vi "Field Draw Field(circular).vi"(6 "Lado,radius, stretch":i32[](array[numeric]), 8 "new picture in":picture, 9 "Offset":cluster{"Width":dbl, "Height":dbl}, 10 "Scale":dbl, 11 "Field Size":T2) -> (0 "new picture out":picture, 1 "Offset Out":cluster{"Width":dbl, "Height":dbl}, 2 "Scale Out":dbl)   [LabVIEW 2017]
panel:
  in  "left":i16=1
  in  "rect":T1
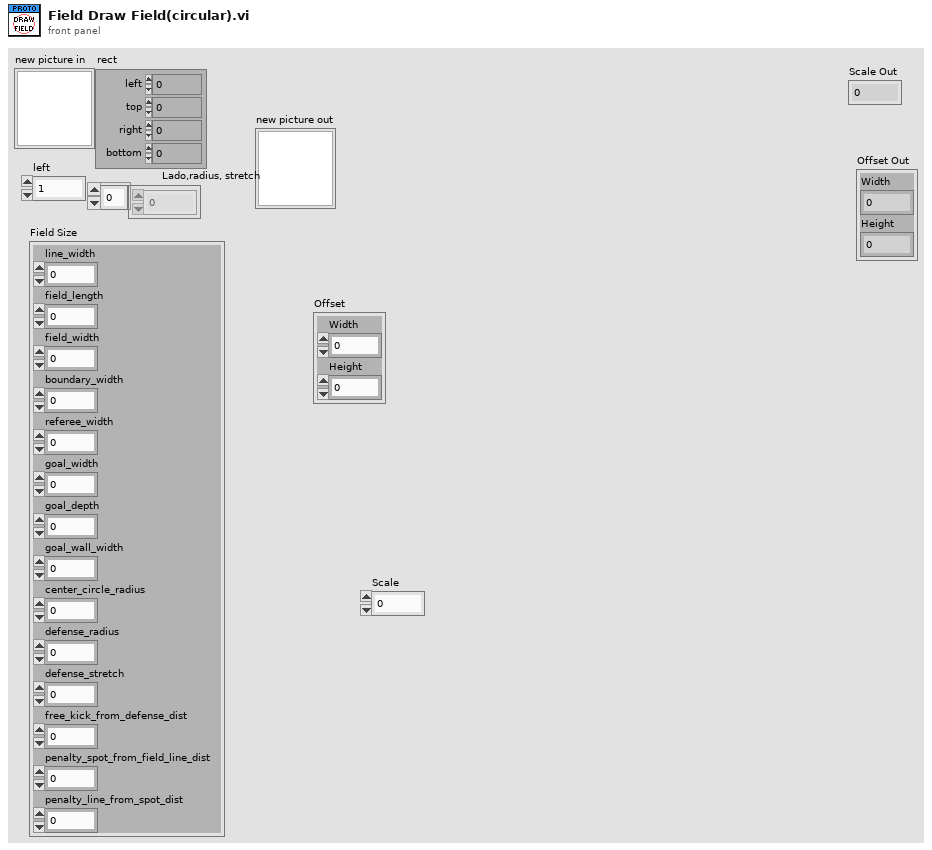
[diagram p1: front panel]
types:
  T1 = cluster{"left":i16, "top":i16, "right":i16, "bottom":i16}
  T2 = cluster{"line_width":u32, "field_length":u32, "field_width":u32, "boundary_width":u32, "referee_width":u32, "goal_width":u32, "goal_depth":u32, "goal_wall_width":u32, "center_circle_radius":u32, "defense_radius":u32, "defense_stretch":u32, "free_kick_from_defense_dist":u32, "penalty_spot_from_field_line_dist":u32, "penalty_line_from_spot_dist":u32}
  T3 = cluster{"Width":i16, "Style":enum32{"Solid", "Dash", "Dot", "DashDot", "DashDotDot"}}
  T4 = cluster{"line_width":dbl, "field_length":dbl, "field_width":dbl, "boundary_width":dbl, "referee_width":dbl, "goal_width":dbl, "goal_depth":dbl, "goal_wall_width":dbl, "center_circle_radius":dbl, "defense_radius":dbl, "defense_stretch":dbl, "free_kick_from_defense_dist":dbl, "penalty_spot_from_field_line_dist":dbl, "penalty_line_from_spot_dist":dbl}
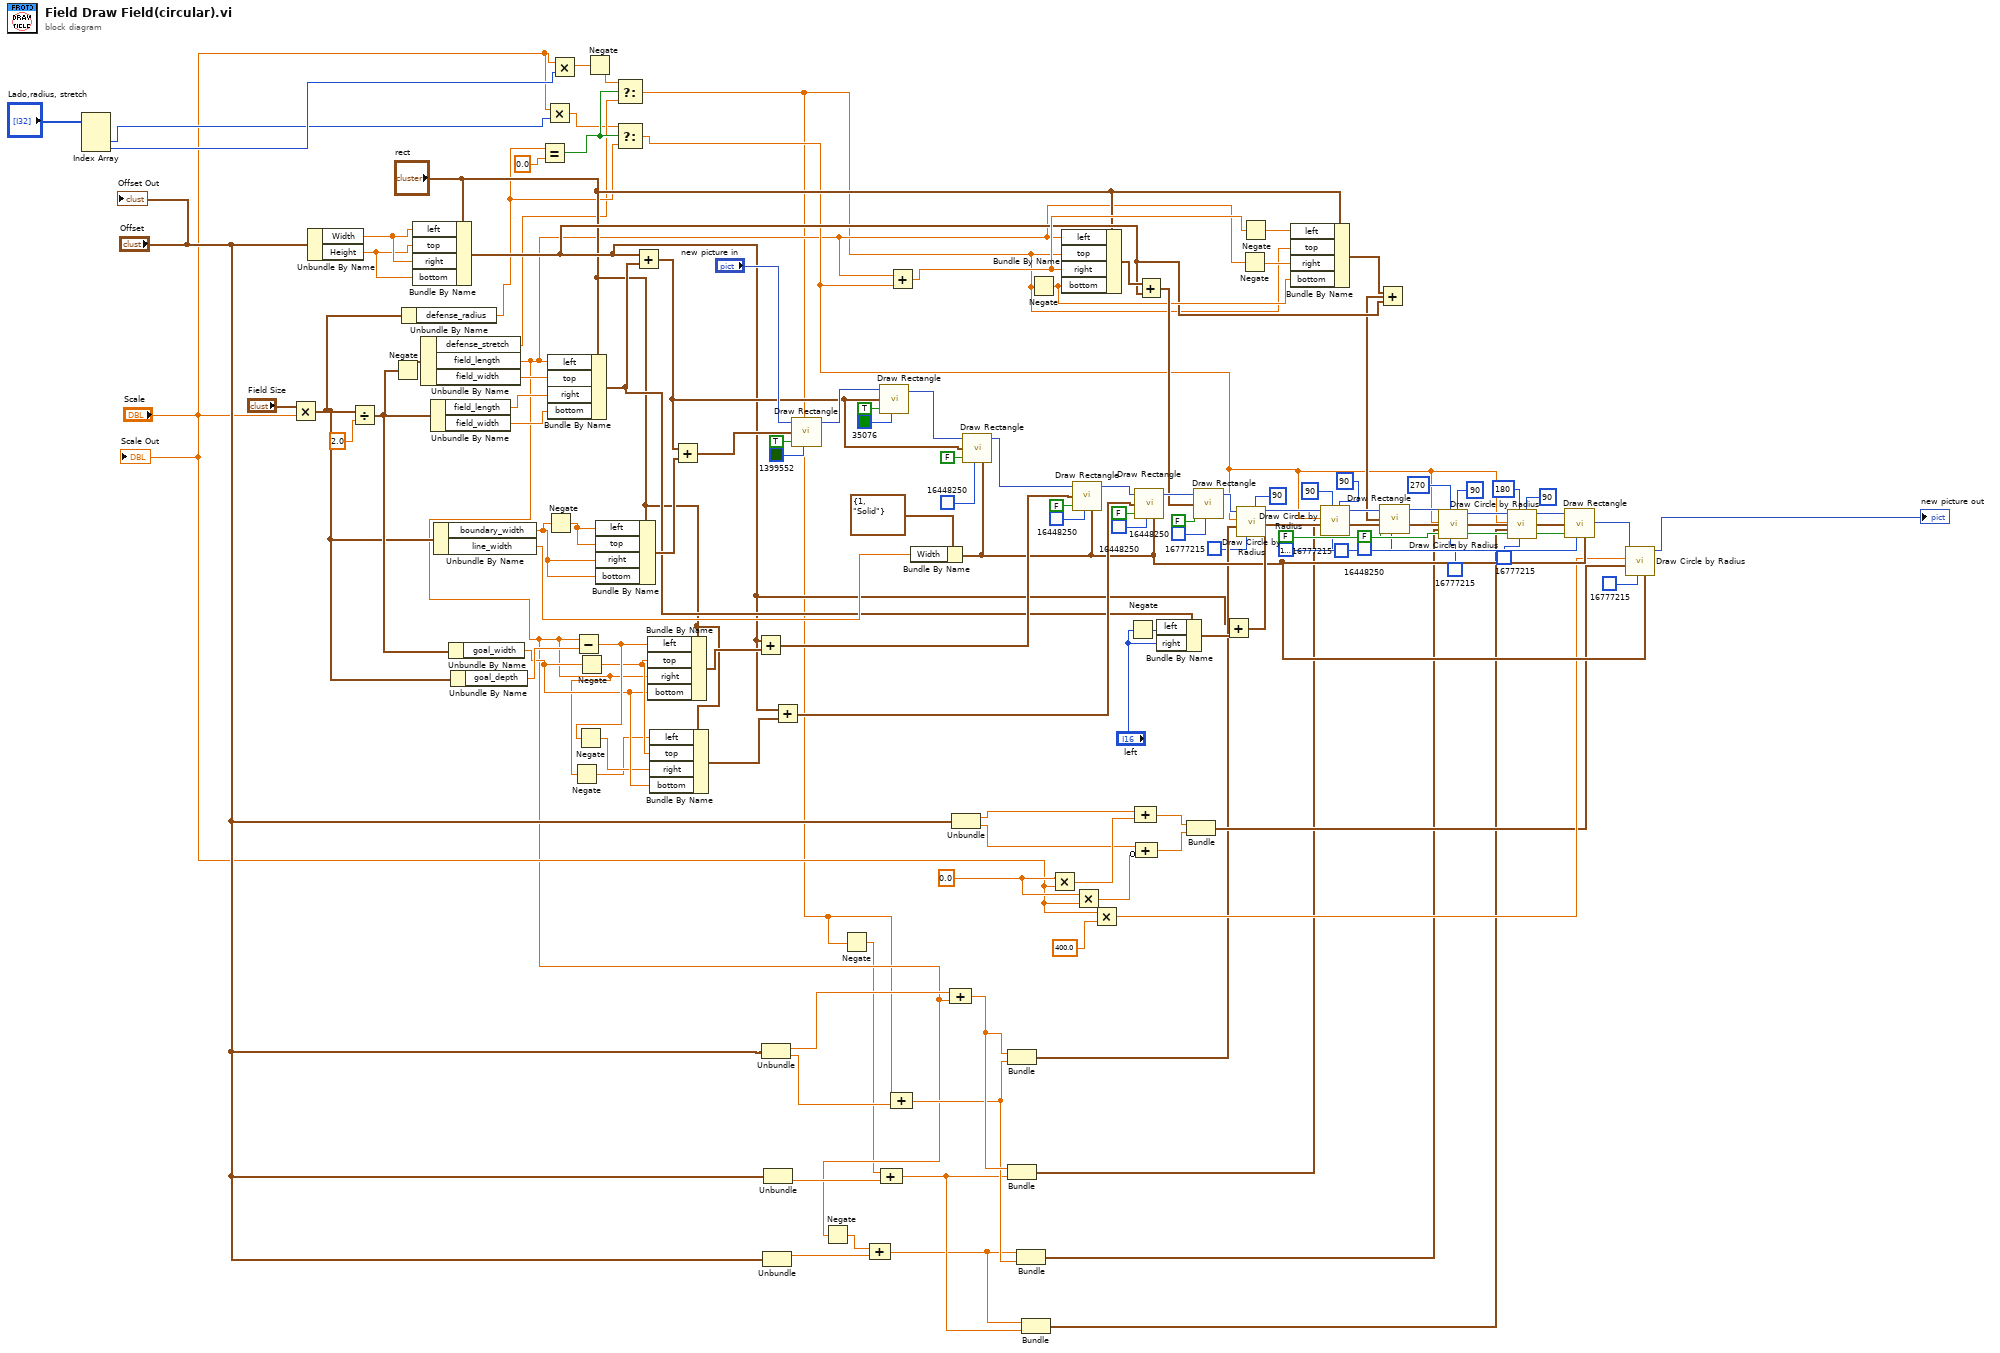
[diagram p0: block diagram]
diagram:
  w64 = 0.0 ("x")
  n1 = Index Array(array="Lado,radius, stretch") -> (element #2=w9:i32, element #3=w10:i32)  [unwired: 3 in, 1 out]
  n2 = Multiply(x="Field Size", y="Scale") -> (x*y=w63:T4)
  n3 = Unbundle By Name("Offset") -> ("Width"=w121:dbl, "Height"=w120:dbl)
  n4 = Divide(x=w63, y=2.0) -> (x/y=w96:T4)
  n5 = Negate(x=w96) -> (-x=w116:T4)
  n6 = Unbundle By Name(w63) -> ("defense_radius"=w13:dbl)
  n7 = Bundle By Name(cluster="rect", "left"=w121, "top"=w120, "right"=w121, "bottom"=w120) -> (w36:T1)
  n8 = Unbundle By Name(w116) -> ("defense_stretch"=w11:dbl, "field_length"=w5:dbl, "field_width"=w119:dbl)
  n9 = Unbundle By Name(w96) -> ("field_length"=w118:dbl, "field_width"=w117:dbl)
  n10 = Unbundle By Name(w63) -> ("boundary_width"=w114:dbl, "line_width"=w103:dbl)
  n11 = Unbundle By Name(w96) -> ("goal_width"=w90:dbl)
  n12 = Unbundle By Name(w63) -> ("goal_depth"=w95:dbl)
  n13 = Equal?(x=w13, y=0.0) -> (x = y?=w12:bool)
  n14 = Multiply(x="Scale", y=w9) -> (x*y=w7:dbl)
  n15 = Negate(x=w114) -> (-x=w115:dbl)
  n16 = Bundle By Name(cluster="rect", "left"=w5, "top"=w119, "right"=w118, "bottom"=w117) -> (w83:T1)
  n17 = Multiply(x="Scale", y=w10) -> (x*y=w2:dbl)
  n18 = Negate(x=w5) -> (-x=w86:dbl)
  n19 = Subtract(x=w5, y=w95) -> (x-y=w92:dbl)
  n20 = Negate(x=w92) -> (-x=w87:dbl)
  n21 = Negate(x=w90) -> (-x=w91:dbl)
  n22 = Negate(x=w2) -> (-x=w1:dbl)
  n23 = Bundle By Name(cluster="rect", "left"=w115, "top"=w115, "right"=w114, "bottom"=w114) -> (w113:T1)
  n24 = Select(t=w1, s=w12, f=w11) -> (s? t:f=w4:dbl)
  n25 = Select(t=w7, s=w12, f=w13) -> (s? t:f=w6:dbl)
  n26 = Add(x=w36, y=w83) -> (x+y=w74:T1)
  n27 = Bundle By Name(cluster="rect", "left"=w92, "top"=w91, "right"=w5, "bottom"=w90) -> (w94:T1)
  n28 = Bundle By Name(cluster="rect", "left"=w86, "top"=w91, "right"=w87, "bottom"=w90) -> (w89:T1)
  n29 = Add(x=w74, y=w113) -> (x+y=w109:T1)
  n30 = Add(x=w36, y=w94) -> (x+y=w93:T1)
  n31 = Unbundle("Offset") -> ("Width"=w57:dbl, "Height"=w55:dbl)
  n32 = Unbundle("Offset") -> ("Width"=w19:dbl)  [unwired: 1 out]
  n33 = Unbundle("Offset") -> ("Height"=w50:dbl)  [unwired: 1 out]
  n34 = Add(x=w36, y=w89) -> (x+y=w88:T1)
  n35 = call <vilib>:"Draw Rectangle.vi"("picture"="new picture in", "rect"=w109, "fill?(F)"=TRUE, "color(black)"=u32 1399552) -> ("new picture"=w108:picture)  [unwired: 5 in]
  n36 = Negate(x=w5) -> (-x=w18:dbl)
  n37 = Negate(x=w4) -> (-x=w3:dbl)
  n38 = Compound Arithmetic op=ADD(w18, w19) -> (w16:dbl)
  n39 = call <vilib>:"Draw Rectangle.vi"("picture"=w108, "rect"=w74, "fill?(F)"=TRUE, "color(black)"=u32 35076) -> ("new picture"=w105:picture)  [unwired: 5 in]
  n40 = Compound Arithmetic op=ADD(w3, w50) -> (w20:dbl)
  n41 = Add(x=w5, y=w6) -> (x+y=w43:dbl)
  n42 = Compound Arithmetic op=ADD(w4, w55) -> (w27:dbl)
  n43 = Bundle By Name(cluster=T3 {"Width"=1, "Style"=enum."Solid"} ("pen"), "Width"=w103) -> (w76:T3)
  n44 = Compound Arithmetic op=ADD(w57, w5) -> (w33:dbl)
  n45 = Unbundle("Offset") -> ("Width"=w72:dbl, "Height"=w69:dbl)
  n46 = call <vilib>:"Draw Rectangle.vi"("picture"=w105, "rect"=w74, "fill?(F)"=FALSE, "color(black)"=u32 16448250, "pen"=w76) -> ("new picture"=w100:picture)  [unwired: 4 in]
  n47 = Bundle(w33, w27) -> (w54:cluster{dbl, dbl})  [unwired: 1 in]
  n48 = Bundle(w33, w20) -> (w47:cluster{dbl, dbl})  [unwired: 1 in]
  n49 = Bundle(w16, w27) -> (w31:cluster{dbl, dbl})  [unwired: 1 in]
  n50 = Bundle(w16, w20) -> (w26:cluster{dbl, dbl})  [unwired: 1 in]
  n51 = Negate(x=w4) -> (-x=w41:dbl)
  n52 = Multiply(x=w64, y="Scale") -> (x*y=w71:dbl)
  n53 = Bundle By Name(cluster="rect", "left"=w5, "top"=w4, "right"=w43, "bottom"=w41) -> (w59:T1)
  n54 = call <vilib>:"Draw Rectangle.vi"("picture"=w100, "rect"=w93, "fill?(F)"=FALSE, "color(black)"=u32 16448250, "pen"=w76) -> ("new picture"=w97:picture)  [unwired: 4 in]
  n55 = Multiply(x=w64, y="Scale") -> (x*y=w68:dbl)
  n56 = Multiply(x="Scale", y=sgl 400.0 ("radius")) -> (x*y=w66:dbl)
  n57 = Negate(x="left") -> (-x=w79:i16)
  n58 = call <vilib>:"Draw Rectangle.vi"("picture"=w97, "rect"=w88, "fill?(F)"=FALSE, "color(black)"=u32 16448250, "pen"=w76) -> ("new picture"=w60:picture)  [unwired: 4 in]
  n59 = Compound Arithmetic op=ADD(w72, w71) -> (w70:dbl)
  n60 = Compound Arithmetic op=ADD(w69, invert w68) -> (w67:dbl)
  n61 = Add(x=w59, y=w36) -> (x+y=w58:T1)
  n62 = Bundle By Name(cluster=w83, "left"=w79, "right"="left") -> (w82:T1)
  n63 = Bundle(w70, w67) -> (w65:cluster{dbl, dbl})  [unwired: 1 in]
  n64 = call <vilib>:"Draw Rectangle.vi"("picture"=w60, "rect"=w58, "fill?(F)"=FALSE, "color(black)"=u32 16448250) -> ("new picture"=w52:picture)  [unwired: 5 in]
  n65 = Add(x=w36, y=w82) -> (x+y=w81:T1)
  n66 = call <vilib>:"Draw Circle by Radius.vi"("arc size(360)"=i16 90, "color(black)"=u32 16777215, "pixel center"=w54, "radius"=w6, "picture"=w52) -> ("new picture"=w49:picture)  [unwired: 6 in]
  n67 = Negate(x=w5) -> (-x=w44:dbl)
  n68 = Negate(x=w43) -> (-x=w42:dbl)
  n69 = Bundle By Name(cluster="rect", "left"=w42, "top"=w4, "right"=w44, "bottom"=w41) -> (w37:T1)
  n70 = call <vilib>:"Draw Circle by Radius.vi"("arc size(360)"=i16 90 ("start angle(0)"), "color(black)"=u32 16777215, "start angle(0)"=i16 90, "pixel center"=w47, "radius"=w6, "picture"=w49) -> ("new picture"=w38:picture)  [unwired: 5 in]
  n71 = Add(x=w37, y=w36) -> (x+y=w35:T1)
  n72 = call <vilib>:"Draw Rectangle.vi"("picture"=w38, "rect"=w35, "fill?(F)"=FALSE, "color(black)"=u32 16448250) -> ("new picture"=w32:picture)  [unwired: 5 in]
  n73 = call <vilib>:"Draw Circle by Radius.vi"("arc size(360)"=i16 90, "color(black)"=u32 16777215, "start angle(0)"=i16 270, "pixel center"=w31, "radius"=w6, "picture"=w32) -> ("new picture"=w24:picture)  [unwired: 5 in]
  n74 = call <vilib>:"Draw Circle by Radius.vi"("arc size(360)"=i16 90, "color(black)"=u32 16777215, "start angle(0)"=i16 180, "pixel center"=w26, "radius"=w6, "picture"=w24) -> ("new picture"=w23:picture)  [unwired: 5 in]
  n75 = call <vilib>:"Draw Rectangle.vi"("picture"=w23, "rect"=w81, "fill?(F)"=FALSE, "color(black)"=u32 16777226, "pen"=w76) -> ("new picture"=w78:picture)  [unwired: 4 in]
  n76 = call <vilib>:"Draw Circle by Radius.vi"("pen"=w76, "color(black)"=u32 16777215, "pixel center"=w65, "radius"=w66, "picture"=w78) -> ("new picture"=→"new picture out":picture)  [unwired: 6 in]
  "Scale Out" <- "Scale"
  "Offset Out" <- "Offset"
